vi "Close.vi"(8 "error in":errorcluster, 11 "Humidity Setpoint in":refnum<class "Humidity Setpoint.lvclass">) -> (0 "error out":errorcluster, 3 "Humidity Setpoint out":refnum<class "Humidity Setpoint.lvclass">)   [LabVIEW 2023, in "Humidity Setpoint.lvclass"]
uses:
  Humidity Setpoint.lvclass
  Humidity Setpoint.lvclass/Humidity Setpoint.ctl
  Parents/Setpoint/Setpoint.lvclass
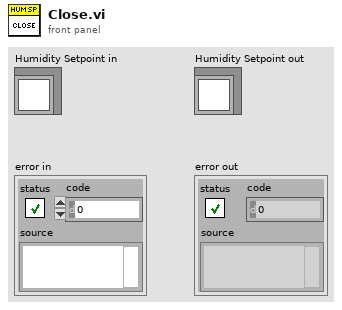
[diagram p1: front panel]
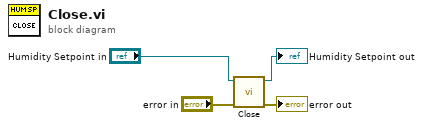
[diagram p0: block diagram]
diagram:
  n1 = call-parent "Close.vi"("error in"="error in", "Setpoint in"="Humidity Setpoint in") -> ("error out"=→"error out":errorcluster, "Setpoint out"=→"Humidity Setpoint out":refnum<class "Humidity Setpoint.lvclass">)  [unwired: 8 in]
